vi "Create Continuous Mask using Formula.vi"(0 "Specification Cluster":cluster{"X":dbl[], "Y":string[]} {"X" format="%.2p"}, 1 "dx":dbl format="%.2p", 2 "x0":dbl=1.0 format="%.2p", 3 "error in (no error)":errorcluster, 4 "Reset":bool) -> (5 "Limit":cluster{"x0":dbl, "dx":dbl, "Y":dbl[]} {"Y" format="%.2p"; "dx" format="%.2p"; "x0" format="%.2p"}, 6 "error out":errorcluster)   [LabVIEW 2020, in "NI_MAPro.lvlib"]
doc: "Creates a continuous or segmented mask in the time domain or in the frequency domain. You can use different instances of this VI to create multiple limits. Wire data to the <B>Specification Cluster</B> input to determine the polymorphic instance to use or manually select the instance."
uses:
  NI_MAPro.lvlib
  NI_Gmath.lvlib
  NI_MABase.lvlib
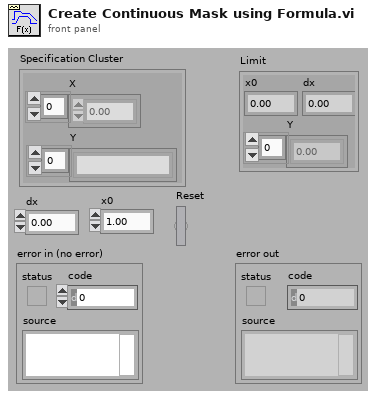
[diagram p1: front panel]
types:
  T1 = enum16{"x < low", "low <= x <= high", "x > high"}
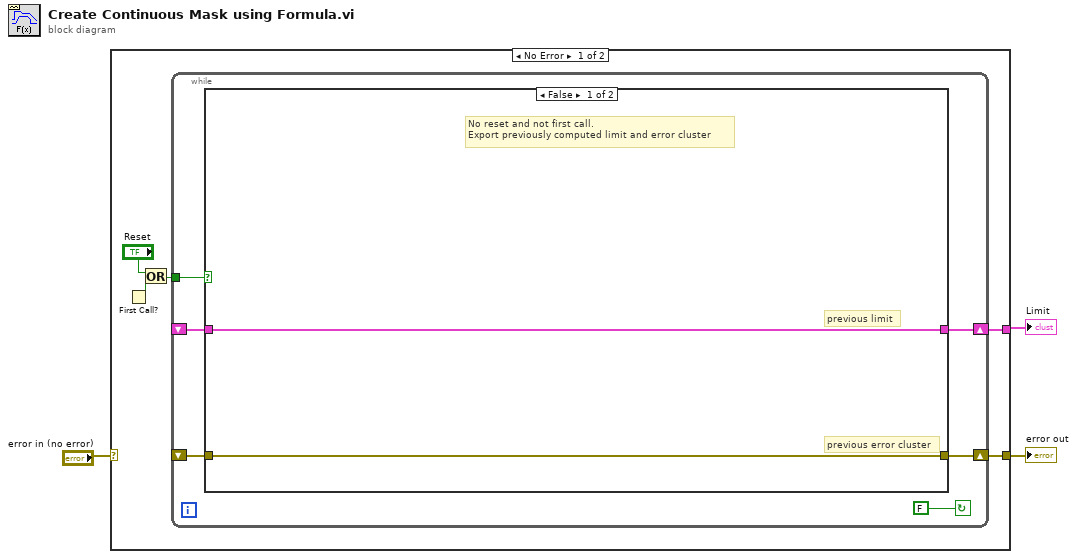
[diagram p0: block diagram]
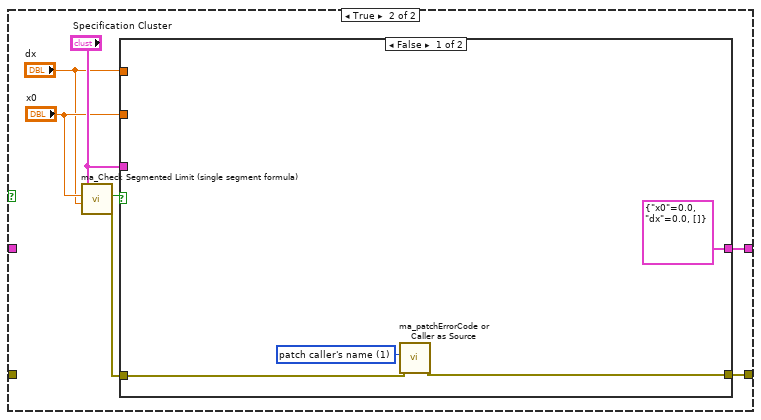
[diagram p2: hidden frame]
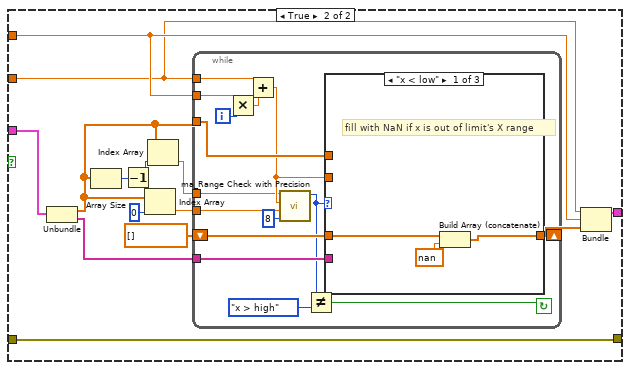
[diagram p3: hidden frame]
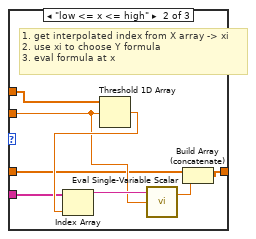
[diagram p4: hidden frame]
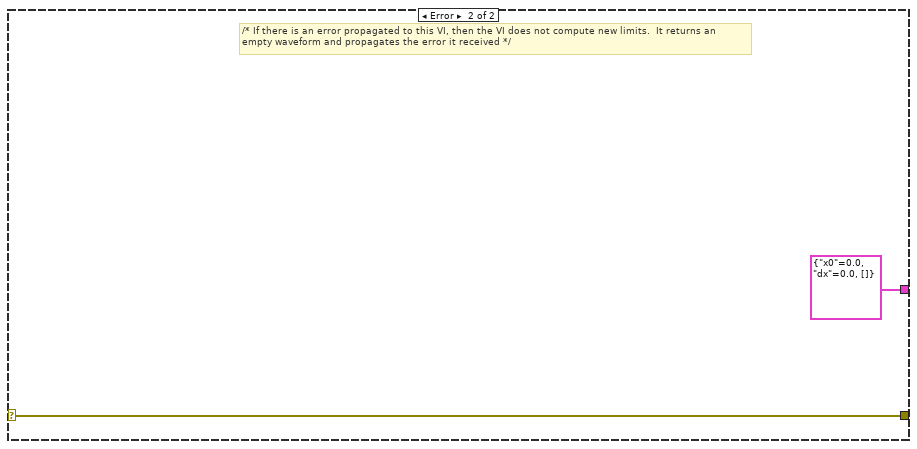
[diagram p6: hidden frame]
diagram:
  n1 = case shown="No Error" "error in (no error)" {
    selector: "error in (no error)" -> [_ w70]
    tunnel: [w8 w70] -> w2
    tunnel: [w7 cluster{"x0":dbl, "dx":dbl, dbl[]} {"x0"=0.0, "dx"=0.0, []}] -> w1
    frame No Error {
      n2 = First Call?() -> (First Call?: T/F=w6:bool)
      n3 = Or(x="Reset", y=w6) -> (x .or. y?=w5:bool)
      n4 = while {
        shift-left: _ -> [w11]
        shift-right: [w13] -> w8
        shift-left: _ -> [w10]
        shift-right: [w14] -> w7
        tunnel: w5 -> [w9]
        stop <- FALSE continue-if-true
        n5 = case shown="False" w9 {
          tunnel: [w16 w23] -> w13
          tunnel: [w15 w22] -> w14
          tunnel: w11 -> [w16 _]
          tunnel: w10 -> [w15 _]
          frame False {
            # "No reset and not first call.\nExport previously computed limit and error cluster"
            # "previous error cluster"
            # "previous limit"
            # "* If Reset is False, the VI does not compute new limits, but uses the one from the previous run.  The limits\nand errors from the previous run are saved in the shift registers */"
          }
          frame True {
            n6 = call "ma_Check Segmented Limit (single segment formula).vi"("Specification Cluster"="Specification Cluster", "x0"="x0", "dx"="dx") -> ("limit spec ok"=w21:bool, "error out"=w20:errorcluster)  [unwired: 6 in]
            n7 = case shown="False" w21 {
              tunnel: [cluster{"x0":dbl, "dx":dbl, dbl[]} {"x0"=0.0, "dx"=0.0, []} w34] -> w22
              tunnel: "dx" -> [_ w31]
              tunnel: w20 -> [w26 w36]
              tunnel: [w25 w36] -> w23
              tunnel: "Specification Cluster" -> [_ w30]
              tunnel: "x0" -> [_ w29]
              frame False {
                w24 = u16 1 items=["patch error code", "patch caller's name"] ("operation")
                n8 = call "ma_patchErrorCode or Caller as Source.vi"("error in (no error)"=w26, "operation"=w24) -> ("error out"=w25:errorcluster)  [unwired: 2 in, 7 out]
              }
              frame True {
                n9 = Unbundle(w30) -> ("X"=w32:dbl[], "Y"=w37:string[])
                n10 = Array Size(array=w32) -> (size(s)=w33:i32)
                n11 = Decrement(x=w33) -> (x-1=w38:i32)
                n12 = Index Array(array=w32, index=0 ("Index")) -> (element=w28:dbl)
                n13 = Index Array(array=w32, index=w38) -> (element=w40:dbl)
                n14 = while {
                  tunnel: w28 -> [w52]
                  tunnel: w32 -> [w53]
                  tunnel: w37 -> [w54]
                  tunnel: w40 -> [w45]
                  shift-left: dbl[] [] -> [w55]
                  shift-right: [w56] -> w35
                  tunnel: w31 -> [w51]
                  tunnel: w29 -> [w49]
                  i -> [w48]
                  stop <- w43 continue-if-true
                  n15 = Multiply(x=w51, y=w48) -> (x*y=w50:dbl)
                  n16 = Add(x=w49, y=w50) -> (x+y=w46:dbl)
                  n17 = call "ma_Range Check with Precision.vi"("precision"=8, "low"=w52, "x"=w46, "high"=w45) -> ("range result"=w42:T1)  [unwired: 7 out]
                  n18 = Not Equal?(x=w42, y=T1."x > high") -> (x != y?=w43:bool)
                  n19 = case shown="\"x < low\"" w42 {
                    tunnel: [w58 w64 w68] -> w56
                    tunnel: w55 -> [w59 w61 w68]
                    tunnel: w54 -> [_ w60 _]
                    tunnel: w53 -> [_ w63 _]
                    tunnel: w46 -> [_ w62 _]
                    frame "x < low" {
                      # "fill with NaN if x is out of limit's X range"
                      n20 = Build Array (concatenate)(w59, nan) -> (w58:dbl[])
                    }
                    frame "low <= x <= high" {
                      # "1. get interpolated index from X array -> xi\n2. use xi to choose Y formula\n3. eval formula at x"
                      n21 = Threshold 1D Array(2:w62, 3:w63) -> (0:w66:dbl)  [unwired: 1 out]
                      n22 = Index Array(array=w60, index=w66) -> (element=w65:string)
                      n23 = call "Eval Single-Variable Scalar.vi"("x value"=w62, "formula"=w65) -> ("y value"=w67:dbl)  [unwired: 1 in, 1 out]
                      n24 = Build Array (concatenate)(w61, w67) -> (w64:dbl[])
                    }
                    frame "x > high", Default {
                    }
                  }
                }
                n25 = Bundle("x0"=w29, "dx"=w31, w35) -> (w34:cluster{"x0":dbl, "dx":dbl, dbl[]})  [unwired: 1 out]
              }
            }
          }
        }
      }
    }
    frame Error {
      # "/* If there is an error propagated to this VI, then the VI does not compute new limits.  It returns an\nempty waveform and propagates the error it received */"
    }
  }
  "error out" <- w2
  "Limit" <- w1
